vi "Add Value to Graph Data.vi"(7 "Graph Data in":cluster{"Array":dbl[], "Array":dbl[]}[](array[cluster]), 8 "Error In":errorcluster, 10 "Value":dbl, 11 "Index":i32) -> (0 "Error Out":errorcluster, 5 "Graph Data out":cluster{"Array":dbl[], "Array":dbl[]}[](array[cluster]))   [LabVIEW 2011]
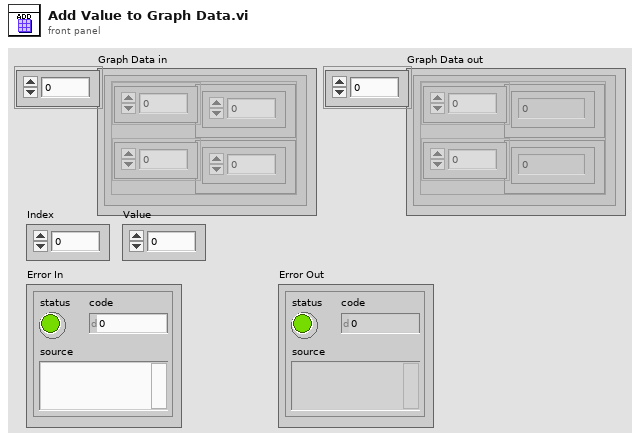
[diagram p1: front panel]
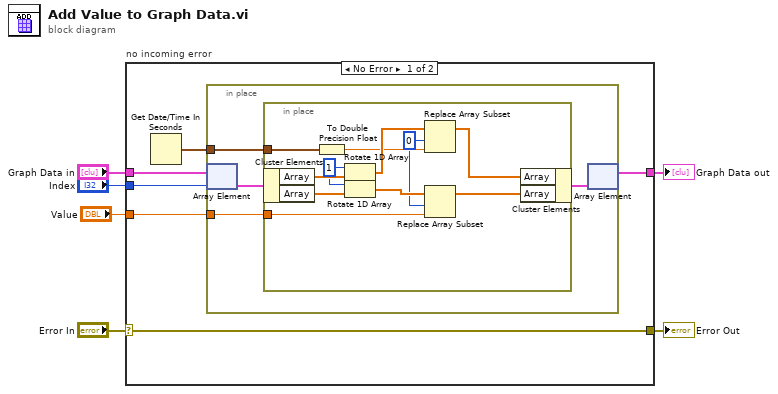
[diagram p0: block diagram]
diagram:
  n1 = case "no incoming error" shown="No Error" "Error In" {
    selector: "Error In" -> [w12 w29]
    tunnel: [w12 w29] -> w5
    tunnel: "Graph Data in" -> [w11 w28]
    tunnel: [w9 w28] -> w3
    tunnel: "Index" -> [w10 _]
    tunnel: "Value" -> [w7 _]
    frame No Error {
      n2 = Get Date/Time In Seconds() -> (seconds since 1Jan1904=w8:timestamp)
      n3 = in-place {
        in-place-border: w8 -> [w14]
        in-place-border: w7 -> [w13]
        n4 = in-place-array #1(w11, w10) -> (w16:cluster{"Array":dbl[], "Array":dbl[]})
        n5 = in-place {
          in-place-border: w14 -> [w23]
          in-place-border: w13 -> [w18]
          w17 = 1 ("n")
          w19 = 0 ("index")
          n6 = in-place-cluster #2(w16) -> ("Array"=w27:dbl[], "Array"=w26:dbl[])
          n7 = To Double Precision Float(number=w23) -> (double precision float=w22:dbl)
          n8 = Rotate 1D Array(1:w27, 2:w17) -> (0:w25:dbl[])
          n9 = Rotate 1D Array(1:w26, 2:w17) -> (0:w21:dbl[])
          n10 = Replace Array Subset(array=w25, new element=w22, index=w19) -> (w24:dbl[])
          n11 = Replace Array Subset(array=w21, new element=w18, index=w19) -> (w20:dbl[])
          n12 = in-place-cluster #2("Array"=w24, "Array"=w20) -> (w15:cluster{"Array":dbl[], "Array":dbl[]})
        }
        n13 = in-place-array #1(w15) -> (w9:cluster{"Array":dbl[], "Array":dbl[]}[])  [unwired: 1 out]
      }
    }
    frame Error {
    }
  }
  "Error Out" <- w5
  "Graph Data out" <- w3
